vi "MoveParameterInit.vi"(8 "error in (no error)":errorcluster, 11 "Position":T1) -> (0 "Error Out":errorcluster)   [LabVIEW 2016, in "SeqProcessor.lvlib"]
uses:
  SeqProcessor.lvlib
  Parameter/controls/Position.ctl
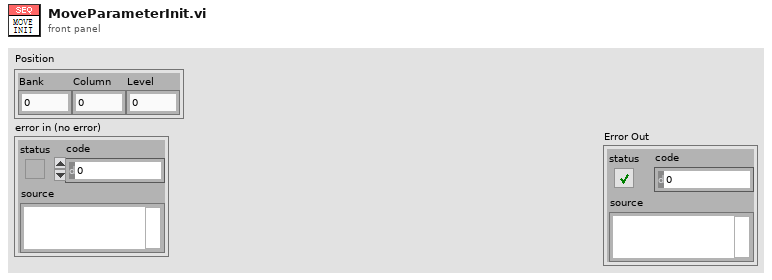
[diagram p1: front panel]
types:
  T1 = typedef "Parameter.lvlib/Position.ctl" = cluster{"Bank":u8, "Column":u8, "Level":u8}
  T2 = typedef "Parameter.lvlib/CasstteCoordinate.ctl" = cluster{"Travel":dbl, "Lift":dbl, "Upper":dbl, "Lower":dbl}
  T3 = typedef "Parameter.lvlib/StockerInfo.ctl" = cluster{"Bank":u8, "Level":u8, "Column":u8, "RotateHPPosition":dbl, "RotateOPPosition":dbl, "LiftUpperLimit":dbl, "LiftLowerLimit":dbl, "ForkOPPositon1":dbl, "ForkOPPosition2":dbl, "TravelLimit":T4, "LiftLimit":T4, "RotateLimit":T4, "ForkLimit":T4}
  T4 = typedef "Parameter.lvlib/LimitPosition.ctl" = cluster{"HPES":dbl, "OPES":dbl}
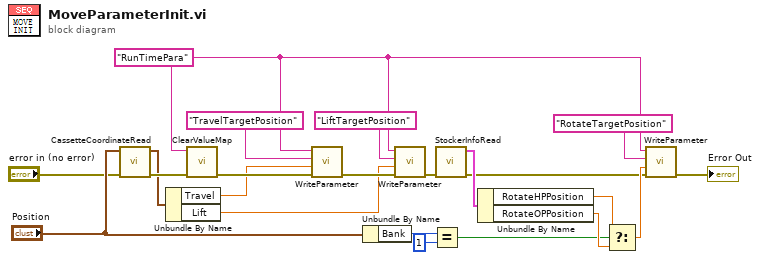
[diagram p0: block diagram]
diagram:
  w17 = "RunTimePara" ("MapName")
  n1 = call "CassetteCoordinateRead.vi"("error in (no error)"="error in (no error)", "Position"="Position") -> ("error out"=w16:errorcluster, "Coordinate"=w15:T2)  [unwired: 8 in]
  n2 = Unbundle By Name(w15) -> ("Travel"=w14:dbl, "Lift"=w13:dbl)
  n3 = call "ClearValueMap.vi"("error in (no error)"=w16, "MapName"=w17) -> ("error out"=w18:errorcluster)  [unwired: 8 in, 1 out]
  n4 = call "WriteParameter.vi"("error in (no error)"=w18, "Value"=w14, "Parameter"="TravelTargetPosition", "MapName"=w17) -> ("Error Out"=w21:errorcluster)  [unwired: 6 in, 1 out]
  n5 = Unbundle By Name("Position") -> ("Bank"=w6:u8)
  n6 = call "WriteParameter.vi"("error in (no error)"=w21, "Value"=w13, "Parameter"="LiftTargetPosition", "MapName"=w17) -> ("Error Out"=w12:errorcluster)  [unwired: 6 in, 1 out]
  n7 = Equal?(x=w6, y=u8 1) -> (x = y?=w4:bool)
  n8 = call "StockerInfoRead.vi"("error in (no error)"=w12) -> ("Error Out"=w7:errorcluster, "StockerInfo"=w11:T3)  [unwired: 8 in, 1 out]
  n9 = Unbundle By Name(w11) -> ("RotateHPPosition"=w10:dbl, "RotateOPPosition"=w9:dbl)
  n10 = Select(t=w10, s=w4, f=w9) -> (s? t:f=w8:dbl)
  n11 = call "WriteParameter.vi"("error in (no error)"=w7, "Value"=w8, "Parameter"="RotateTargetPosition", "MapName"=w17) -> ("Error Out"=→"Error Out":errorcluster)  [unwired: 6 in, 1 out]
